vi "(SubVI) RFID.vi"(1 "Nº Decimal":u32) -> (0 "Nº Binário":string)   [LabVIEW 2010]
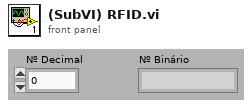
[diagram p1: front panel]
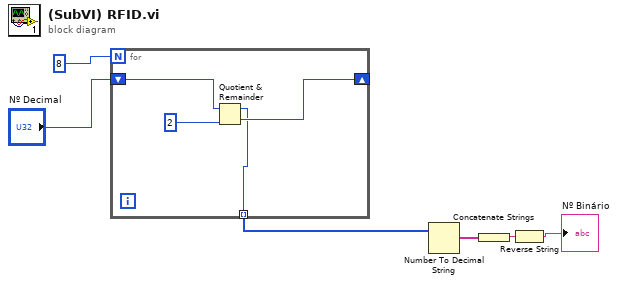
[diagram p0: block diagram]
diagram:
  n1 = for {
    N: 8 -> [_]
    shift-right: [w9] -> _
    shift-left: "Nº Decimal" -> [w8]
    tunnel: [w7] -> w4 mode=indexing
    n2 = Quotient & Remainder(x=w8, y=u32 2) -> (x-y*floor(x/y)=w7:u32, floor(x/y)=w9:u32)
  }
  n3 = Number To Decimal String(number=w4) -> (decimal integer string=w3:string[])  [unwired: 1 in]
  n4 = Concatenate Strings(w3) -> (w5:string)
  n5 = Reverse String(1:w5) -> (0:→"Nº Binário":string)
